vi "Calibartion-UI.vi"(8 "error in (no error)":errorcluster, 11 "Data (in)":T1={"Xml Path?"=path "", "Calib_List"=[], "Calibration Tbl Value"=-1, "Tbl_Size"=4294967295, "Parameter List"=[]}) -> (0 "error out":errorcluster, 3 "Data (out)":T1={"Xml Path?"=path "", "Calib_List"=[], "Calibration Tbl Value"=-1, "Tbl_Size"=4294967295, "Parameter List"=[]})   [LabVIEW 2010]
uses:
  Calibration_UI_Data.ctl
  Calibration dates.ctl
  <userlib>/_VIE Internal Reuse Library/_vie_lib_queued_message_handler.llb/VIE.Module.Queued Message Handler.enqueue.State.PolyChild.QueuedMessageHandler.vi
  <userlib>/_VIE Internal Reuse Library/_vie_lib_queued_message_handler.llb/VIE.Module.Queued Message Handler.[enqueue].State.PolyChild.QueuedMessageHandler.vi
  <vilib>/Utility/xml.llb/Write to XML File(string).vi
  <vilib>/Utility/xml.llb/Read From XML File(string).vi
  <userlib>/_VIE Internal Reuse Library/_vie_lib_queued_message_handler.llb/VIE.Module.Queued Message Handler.QueuedMessageHandler.dqGOOPClass.lvlib
panel:
  out "Cal Due Date":string="MM/DD/YY"
  in  "Calibration Details":i32(listbox)
  in  "Calibrate All":bool
  out "Name.Minor.Foreground":string="Automated Test Execution Software"
  out "Name.Major.Foreground":string="ATES"
  out "Name.Major.Background":string="ATES"
  out "Name.Minor.Background":string="Automated Test Execution Software"
  in  "Calibration Utility":bool
  out "IPG Calibration Status":bool
  # "(Double Click on the row to calibrate it)"
  # "Use the CVT as a data bus for data that is\nto be accesed outside of the VI.  It can be\nused for data passed around  inside the state\nmachine too, and all local data can be selectively\npurged from the CVT in the \"system.Exit\" state."
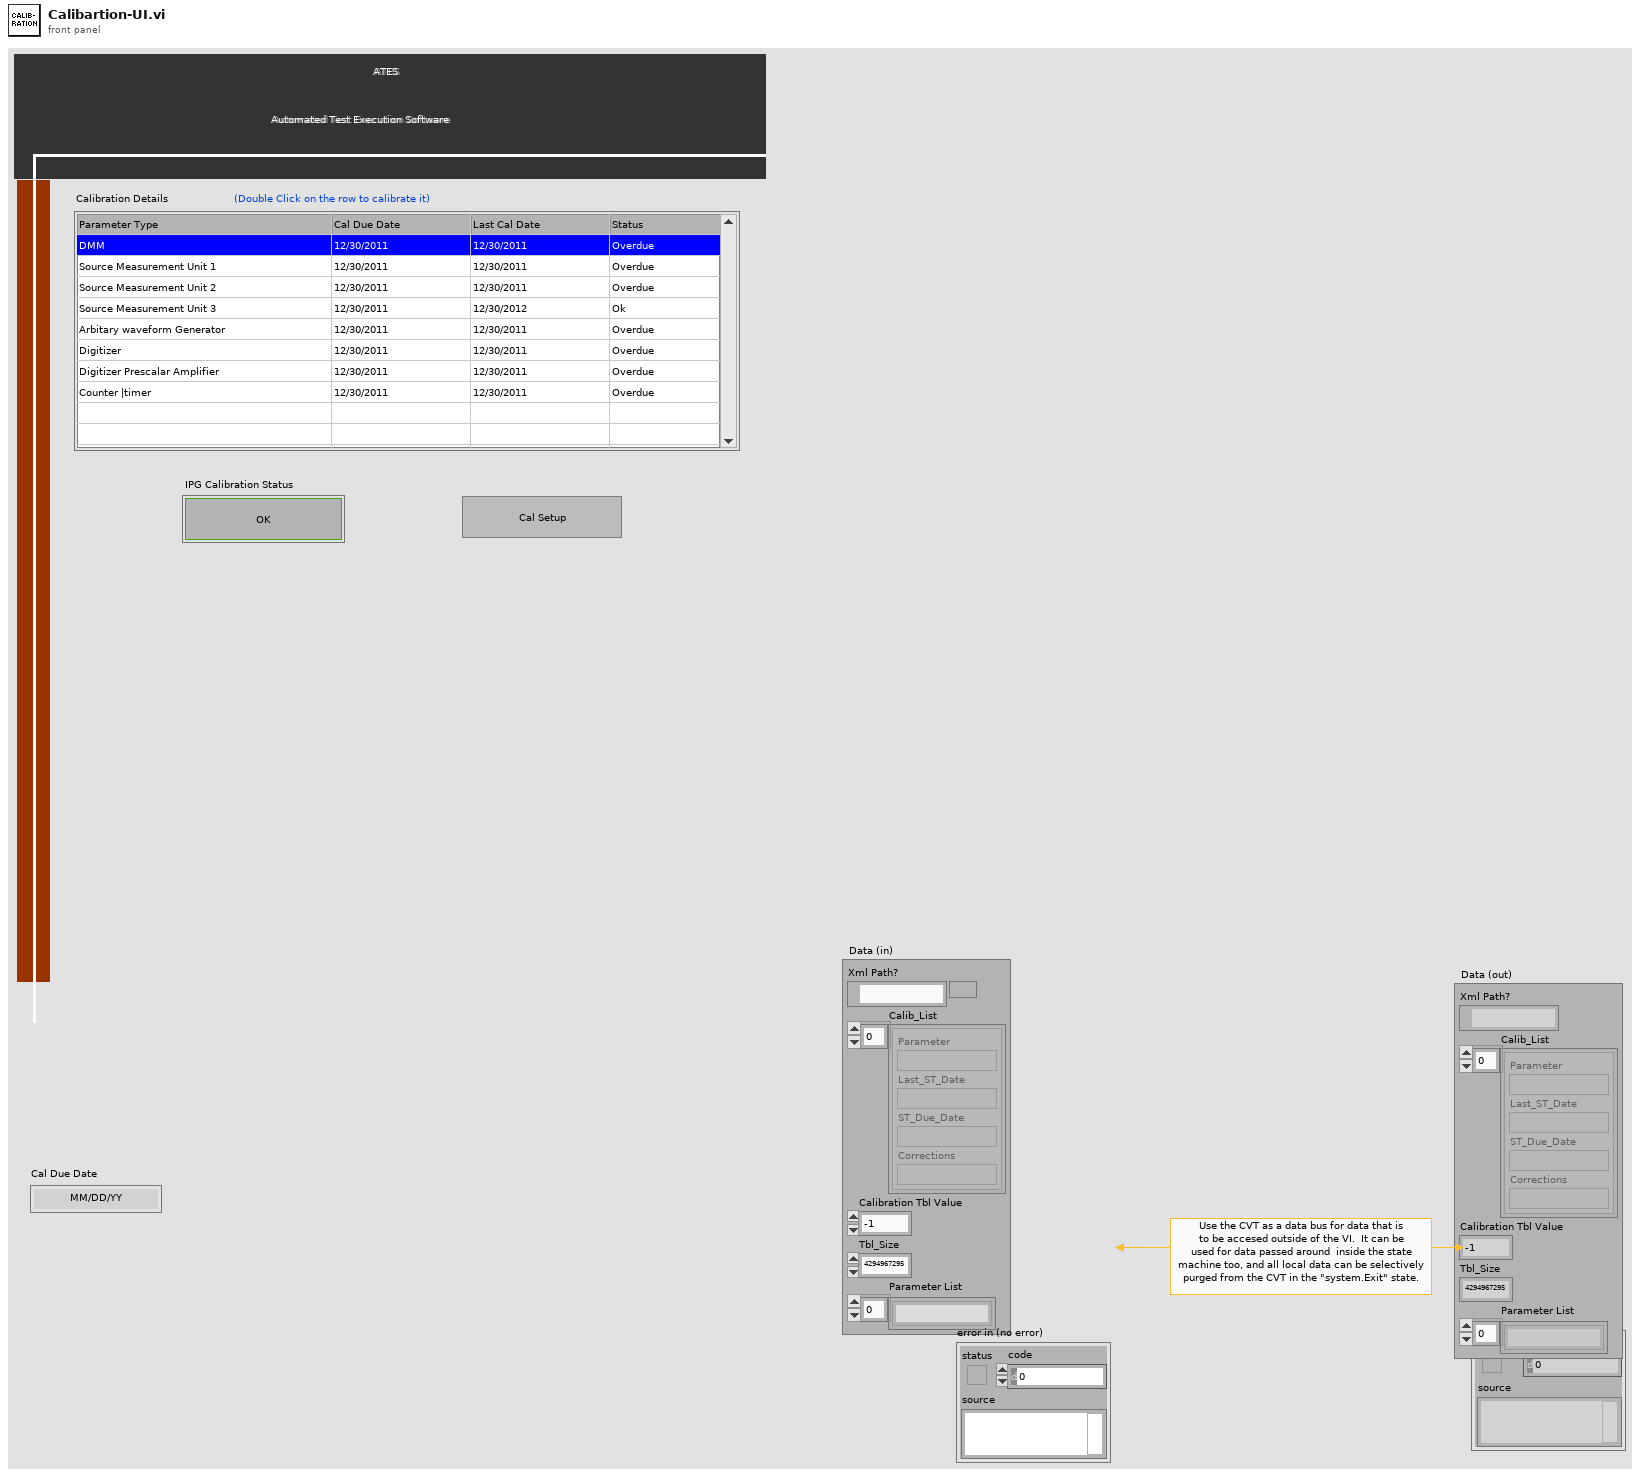
[diagram p1: front panel]
types:
  T1 = typedef "Calibration_UI_Data.ctl" = cluster{"Xml Path?":path, "Calib_List":T2[], "Calibration Tbl Value":i32, "Tbl_Size":u32, "Parameter List":string[]}
  T2 = typedef "Calibration dates.ctl" = cluster{"Parameter":string, "Last_ST_Date":string, "ST_Due_Date":string, "Corrections":string}
  T3 = enum16{"open", "replace", "create", "open or create", "replace or create", "replace or create with confirmation"}
  T4 = enum32{"invalid app kind", "Development System", "Run Time System", "Student Edition", "Embedded LabVIEW", "Evaluation", "Custom"}
  T5 = typedef "VIE.Module.Queued Message Handler.QueuedMessageHandler.dqGOOPClass.lvlib/VIE.Module.Queued Message Handler.dqClass_ObjectReference.ctl" = refnum<k1>
  T6 = typedef "LVPoint32TypeDef.ctl" = cluster{"Horizontal":i32, "Vertical":i32}
  T7 = typedef "LVRowAndColumnTypeDef.ctl" = cluster{"Row":i32, "Column":i32}
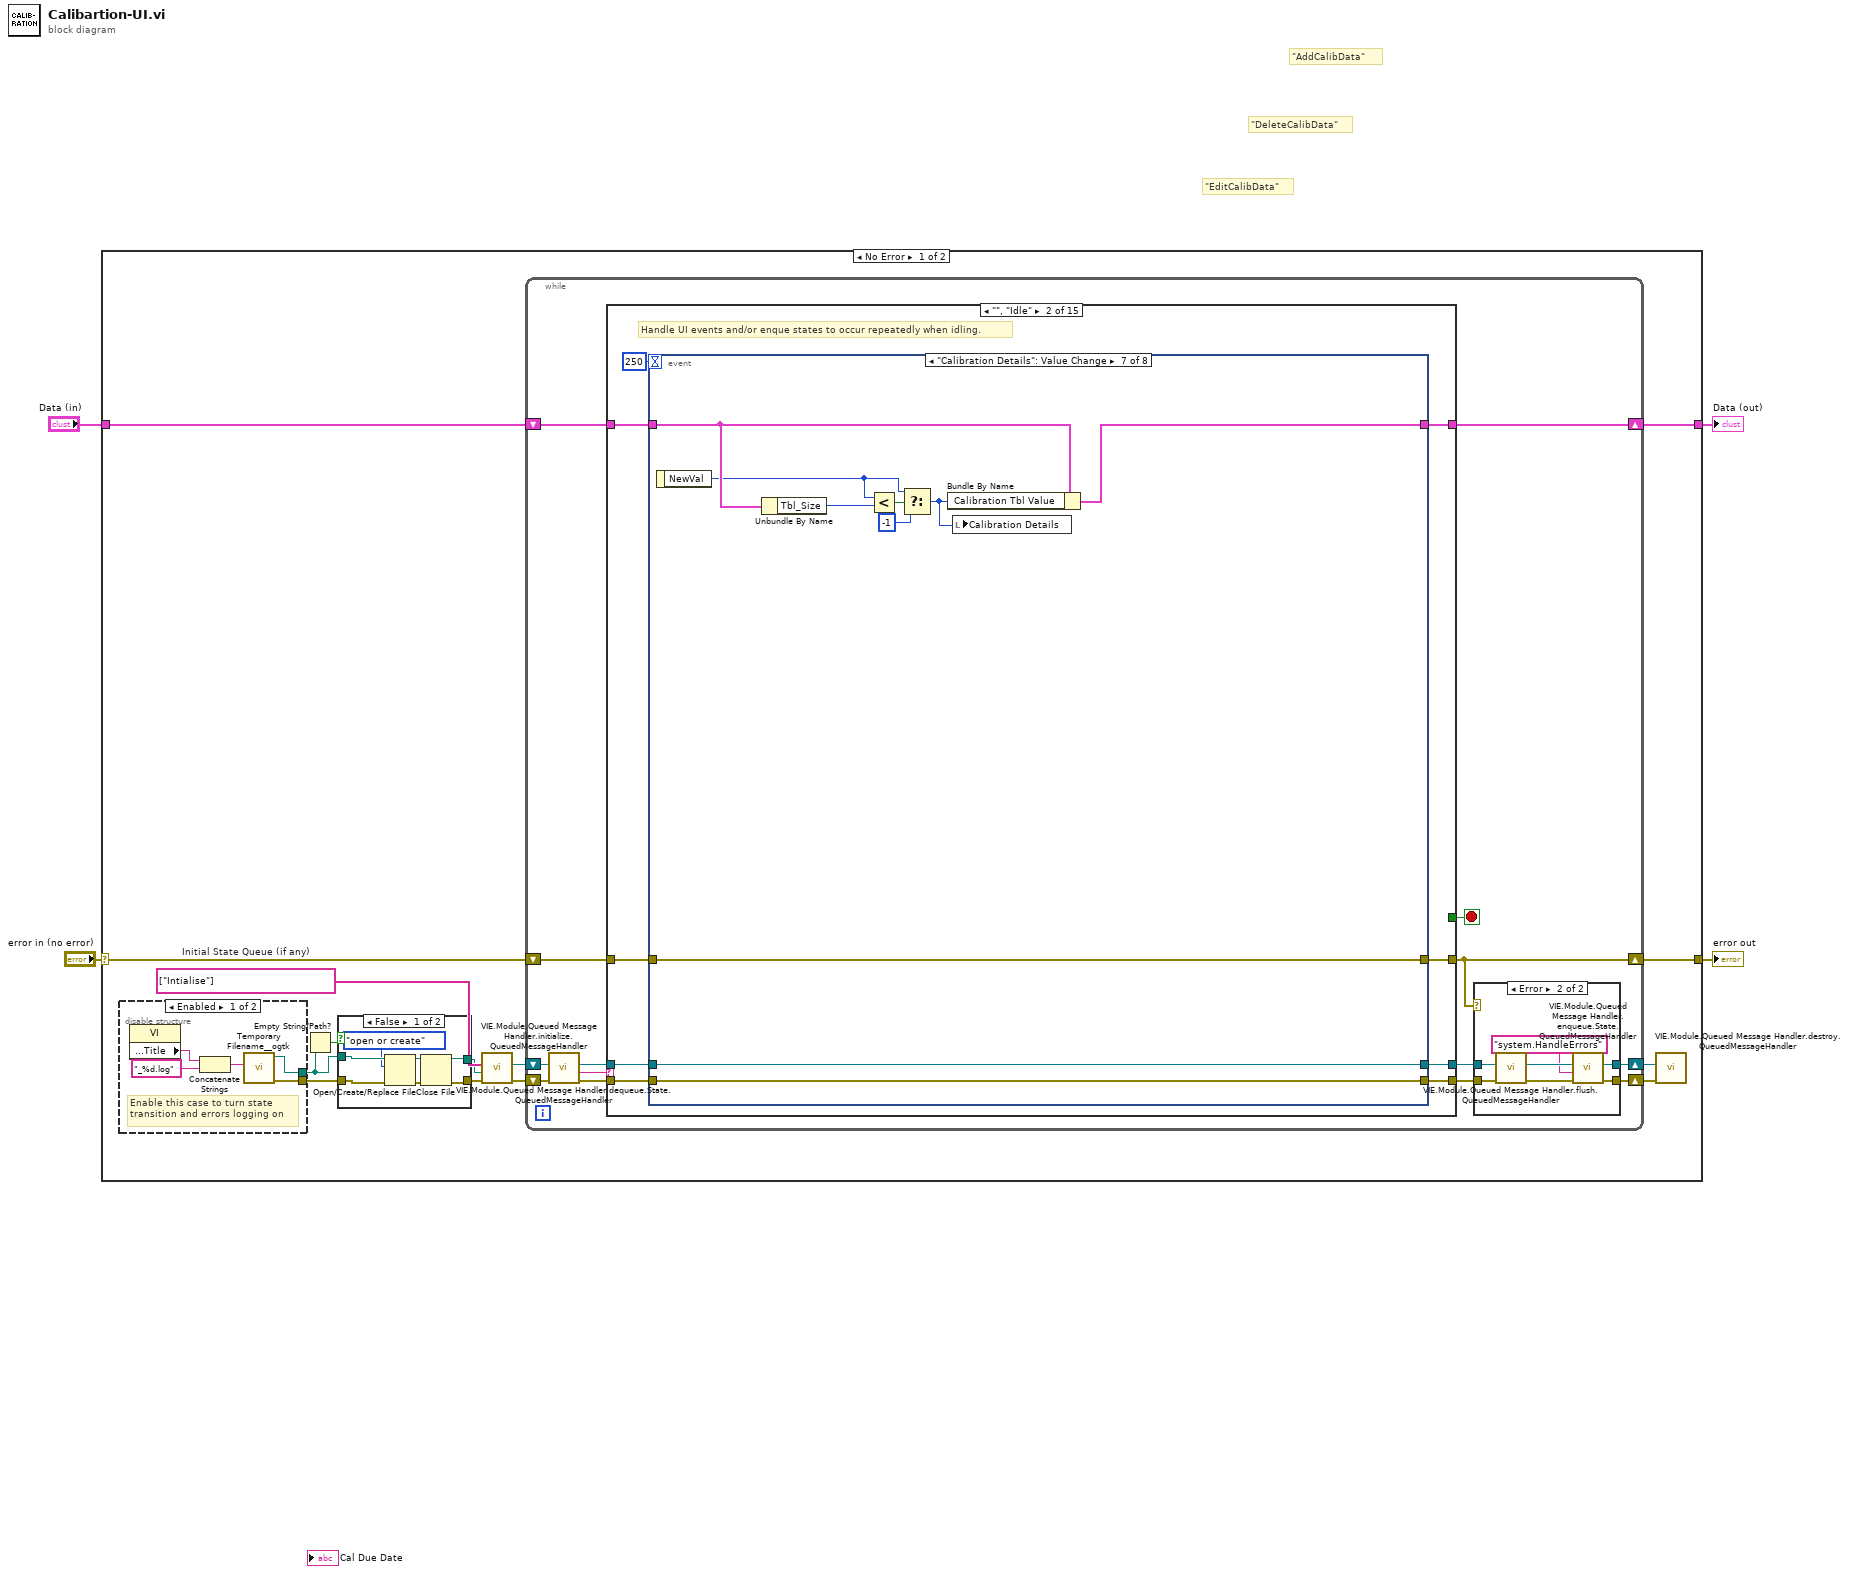
[diagram p0: block diagram]
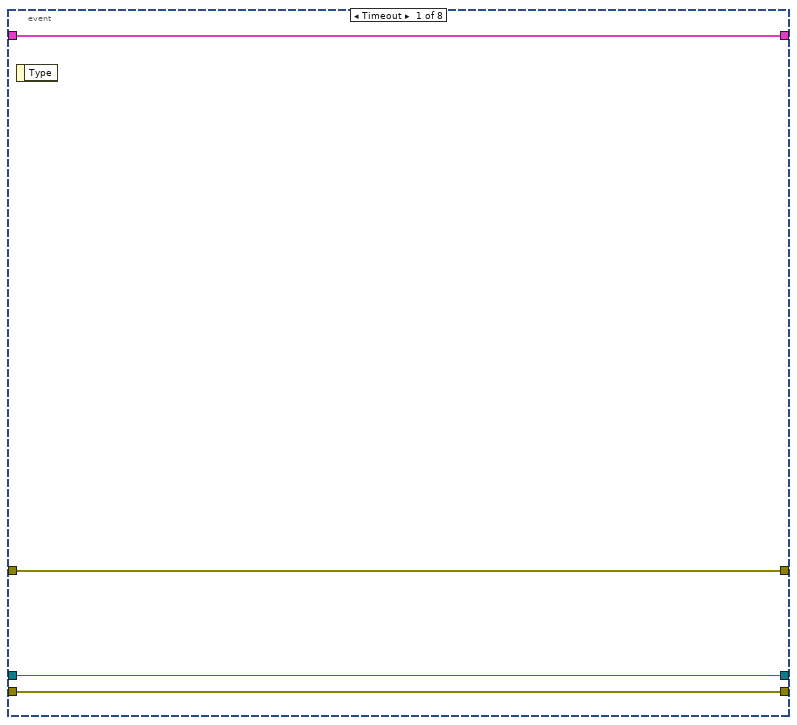
[diagram p6: hidden frame]
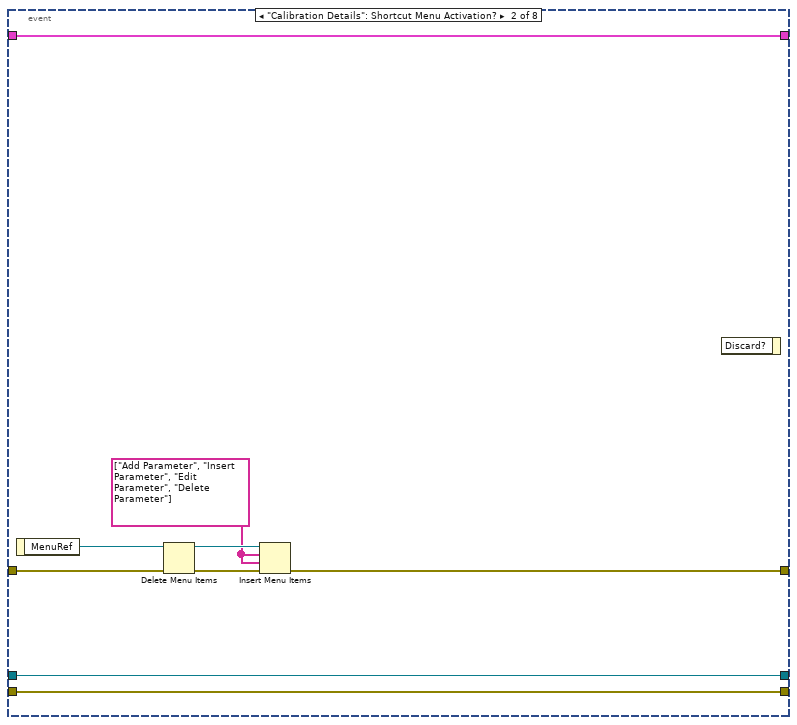
[diagram p7: hidden frame]
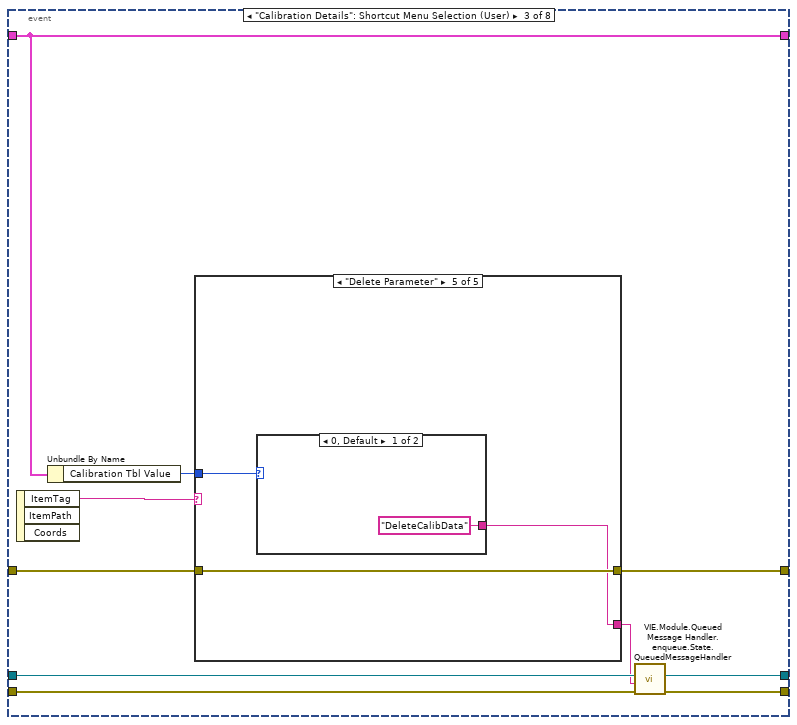
[diagram p8: hidden frame]
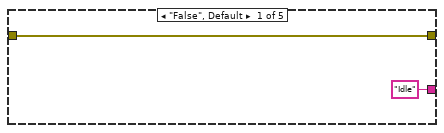
[diagram p9: hidden frame]
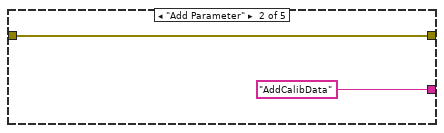
[diagram p10: hidden frame]
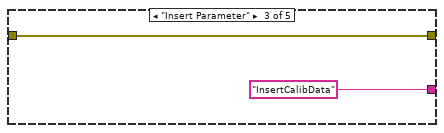
[diagram p11: hidden frame]
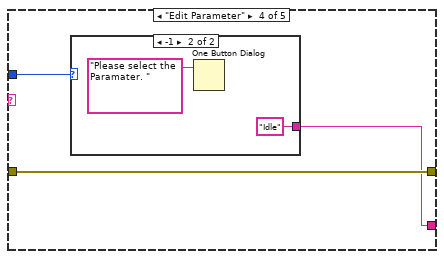
[diagram p12: hidden frame]
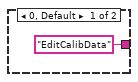
[diagram p13: hidden frame]
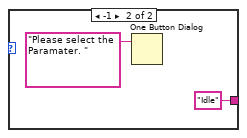
[diagram p14: hidden frame]
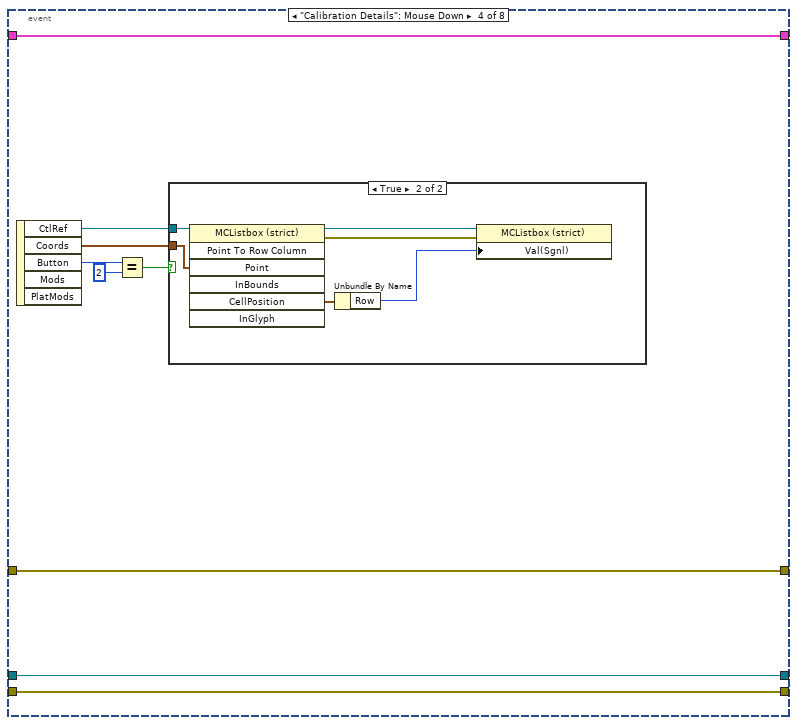
[diagram p15: hidden frame]
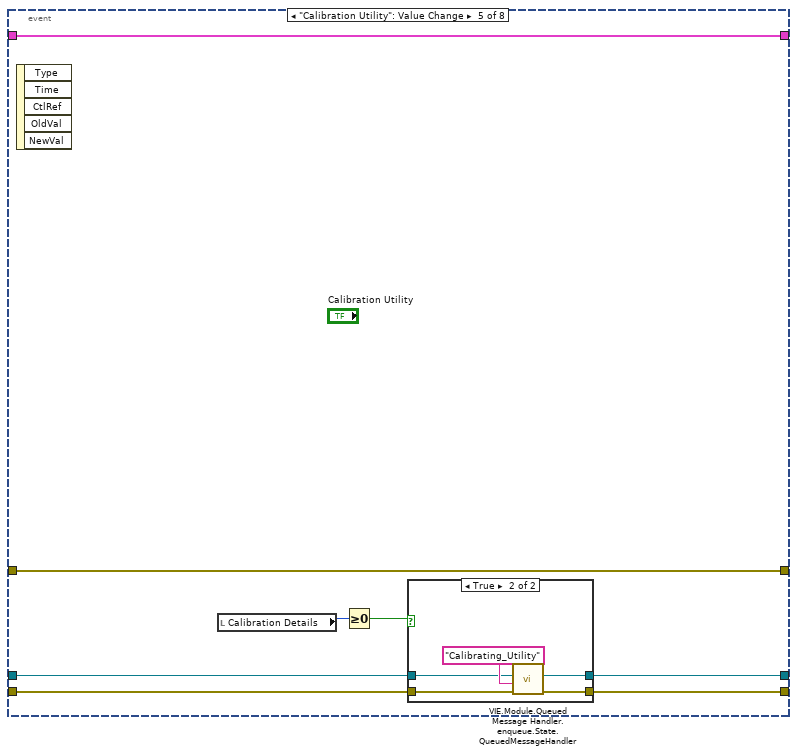
[diagram p17: hidden frame]
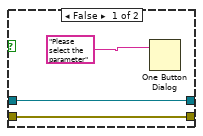
[diagram p18: hidden frame]
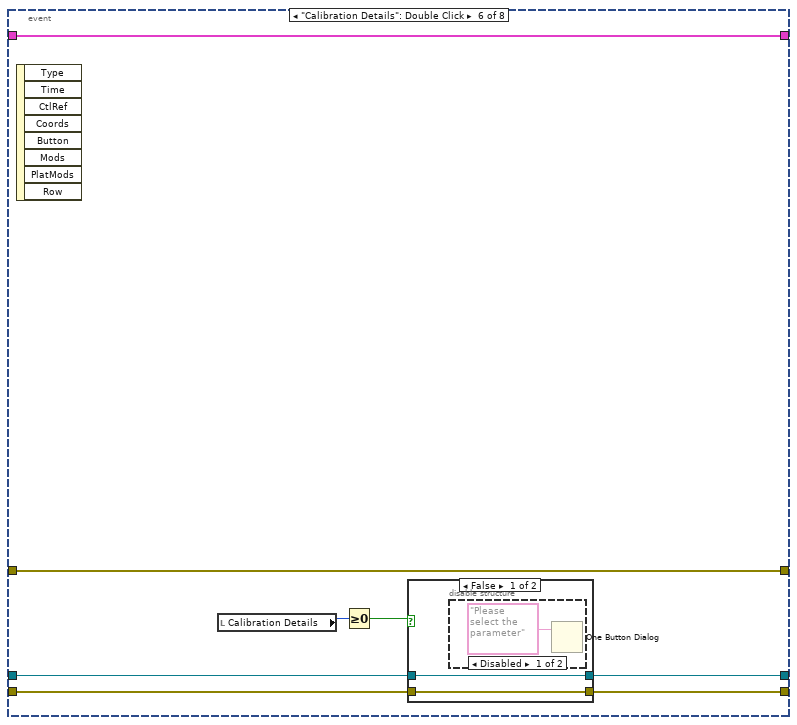
[diagram p19: hidden frame]
diagram:
  # "\"AddCalibData\""
  # "\"EditCalibData\""
  # "\"DeleteCalibData\""
  n1 = case shown="No Error" "error in (no error)" {
    selector: "error in (no error)" -> [w13 w462]
    tunnel: [w12 w462] -> w3
    tunnel: "Data (in)" -> [w10 w461]
    tunnel: [w14 w461] -> w1
    frame No Error {
      w11 = string[] ["Intialise"]  # Initial State Queue (if any)
      n2 = disable-structure shown="Enabled" {
        disable-tunnel: [w29 _] -> w8
        disable-tunnel: [w28 _] -> w9
        frame Enabled {
          # "Enable this case to turn state\ntransition and errors logging on"
          n3 = property class="VI"() -> ("Front Panel.Title"=w30:string)  [unwired: 2 in, 2 out]
          n4 = Concatenate Strings(w30, "_%d.log" ("string")) -> (w32:string)
          n5 = call <userlib>:"Temporary Filename__ogtk.vi"("pattern (lvtemp%d.tmp)"=w32) -> ("error out"=w29:errorcluster, "file in tmp dir"=w28:path)  [unwired: 5 in]
        }
        frame Disabled {
          # "Enable this case to turn state\ntransition and errors logging off"
        }
      }
      n6 = Empty String/Path?(string/path=w9) -> (empty?=w5:bool)
      n7 = case shown="False" w5 {
        tunnel: w8 -> [w25 w27]
        tunnel: [w20 w27] -> w7
        tunnel: w9 -> [w24 w26]
        tunnel: [w19 w26] -> w6
        frame False {
          n8 = Open/Create/Replace File(file path (use dialog)=w24, error in=w25, operation (0:open)=T3."open or create") -> (refnum out=w22:refnum<file>, error out=w21:errorcluster)  [unwired: 3 in, 1 out]
          n9 = Close File(refnum=w22, error in=w21) -> (path=w19:path, error out=w20:errorcluster)
        }
        frame True {
        }
      }
      n10 = call <userlib>:"VIE.Module.Queued Message Handler.initialize.QueuedMessageHandler.vi"("error in (no error)"=w7, "State Queue Log FilePath (\"\" = Do Not Log)"=w6, "Initial State Queue (empty)"=w11) -> ("error out"=w18:errorcluster, "QueuedMessageHandler.dqGOOPClass (out)"=w15:T5)  [unwired: 7 in]
      n11 = while {
        shift-right: [w35] -> w17
        shift-left: w18 -> [w43]
        shift-right: [w40] -> w14
        shift-left: w10 -> [w41]
        shift-right: [w38] -> w12
        shift-left: w13 -> [w39]
        shift-right: [w34] -> w16
        shift-left: w15 -> [w46]
        stop <- w33 stop-if-true
        n12 = call <userlib>:"VIE.Module.Queued Message Handler.dequeue.State.QueuedMessageHandler.vi"("error in (no error)"=w43, "QueuedMessageHandler.dqGOOPClass (in)"=w46) -> ("error out"=w44:errorcluster, "State Dequeued"=w42:string, "QueuedMessageHandler.dqGOOPClass (out)"=w45:T5)  [unwired: 7 in]
        n13 = case shown="\"\", \"Idle\"" w42 {
          selector: w42 -> [_ _ _ _ _ _ _ _ _ _ _ _ w413 _ _]
          tunnel: w44 -> [w56 w66 w179 w235 w267 w289 w314 w348 w371 w383 w400 w407 w412 w430 w454]
          tunnel: [w56 w61 w188 w247 w276 w300 w325 w356 w373 w381 w400 w407 w412 w421 w454] -> w37
          tunnel: w45 -> [w57 w65 w180 w236 w268 w290 w315 w350 w370 w384 w401 w408 w411 w431 w455]
          tunnel: [w57 w62 w187 w246 w275 w299 w324 w355 w372 w382 w401 w408 w411 w422 w455] -> w36
          tunnel: w41 -> [w59 w68 w183 w239 w271 w293 w318 w344 w368 w385 w392 w410 w420 w434 w453]
          tunnel: [w59 w64 w182 w238 w270 w292 w317 w344 w367 w385 w393 w410 w420 w434 w453] -> w40
          tunnel: w39 -> [w58 w67 w178 w245 w274 w298 w323 w354 w362 w379 w398 w409 w415 w432 w448]
          tunnel: [w58 w63 w186 w244 w273 w297 w322 w353 w357 w379 w397 w409 w414 w425 w447] -> w38
          tunnel: [_ _ _ _ _ _ _ _ _ _ _ _ _ _ TRUE] -> w33
          frame "---- Custom States --------------------------" {
            # "Do not put any code in here - this is a case divider, and is not a valid state, so any code here will not be executed."
          }
          frame "", "Idle" {
            # "Handle UI events and/or enque states to occur repeatedly when idling."
            n14 = event shown="[6] \"Calibration Details\": Value Change" {
              selector: _ -> [_ _ _ _ _ _ _ _]
              dyn-events: _ -> [_ _ _ _ _ _ _ _]
              timeout: 250 -> [_ _ _ _ _ _ _ _]
              tunnel: w68 -> [w72 w81 w83 w118 w132 w148 w162 w174]
              tunnel: w67 -> [w69 w74 w91 w115 w131 w147 w166 w173]
              tunnel: w66 -> [w70 w79 w88 w116 w130 w146 w165 w169]
              tunnel: w65 -> [w71 w80 w86 w117 w128 w144 w164 w171]
              tunnel: [w72 w81 w83 w118 w132 w148 w163 w174] -> w64
              tunnel: [w69 w73 w90 w115 w131 w147 w166 w173] -> w63
              tunnel: [w71 w80 w85 w117 w127 w143 w164 w170] -> w62
              tunnel: [w70 w79 w87 w116 w129 w145 w165 w168] -> w61
              event Timeout {
                n15 = event-data() -> ()  [unwired: 1 in, 1 out]
              }
              event "Calibration Details": Shortcut Menu Activation? {
                w75 = string[] ["Add Parameter", "Insert Parameter", "Edit Parameter", "Delete Parameter"]
                n16 = event-data() -> ("MenuRef"=w76:refnum<k9>)  [unwired: 1 in]
                n17 = Delete Menu Items(6:w74, 9:w76) -> (0:w77:errorcluster, 3:w78:refnum<k9>)  [unwired: 2 in]
                n18 = Insert Menu Items(6:w77, 7:w75, 8:w75, 9:w78) -> (0:w73:errorcluster)  [unwired: 2 in, 2 out]
                n19 = event-data() -> ()  [unwired: 2 in, 1 out]
              }
              event "Calibration Details": Shortcut Menu Selection (User) {
                n20 = event-data() -> ("ItemTag"=w89:string)  [unwired: 1 in, 2 out]
                n21 = Unbundle By Name(w83) -> ("Calibration Tbl Value"=w82:i32)
                n22 = case shown="\"Delete Parameter\"" w89 {
                  tunnel: w91 -> [w93 w95 w97 w100 w106]
                  tunnel: [w93 w95 w97 w100 w106] -> w90
                  tunnel: ["Idle" ("State to Enqueue") "AddCalibData" ("State to Enqueue") "InsertCalibData" ("State to Enqueue") w98 w104] -> w84
                  tunnel: w82 -> [_ _ _ w99 w105]
                  frame "False", Default {
                  }
                  frame "Add Parameter" {
                  }
                  frame "Insert Parameter" {
                  }
                  frame "Edit Parameter" {
                    n23 = case shown="-1" w99 {
                      tunnel: ["EditCalibData" ("State to Enqueue") "Idle" ("State to Enqueue")] -> w98
                      frame 0, Default {
                      }
                      frame -1 {
                        n24 = One Button Dialog(message="Please select the Paramater. ") -> ()  [unwired: 1 in, 1 out]
                      }
                    }
                  }
                  frame "Delete Parameter" {
                    n25 = case shown="0, Default" w105 {
                      tunnel: ["DeleteCalibData" ("State to Enqueue") "Idle" ("State to Enqueue")] -> w104
                      frame 0, Default {
                      }
                      frame -1 {
                        n26 = One Button Dialog(message="Please select the Paramater. ") -> ()  [unwired: 1 in, 1 out]
                      }
                    }
                  }
                }
                n27 = call-poly <userlib>:"VIE.Module.Queued Message Handler.enqueue.State.QueuedMessageHandler.vi"("error in (no error)"=w88, "State to Enqueue"=w84, "QueuedMessageHandler.dqGOOPClass (in)"=w86) -> ("error out"=w87:errorcluster, "QueuedMessageHandler.dqGOOPClass (out)"=w85:T5)  [unwired: 7 in]
              }
              event "Calibration Details": Mouse Down {
                n28 = event-data() -> ("CtlRef"=w112:refnum<vi>, "Coords"=w113:T6, "Button"=w111:u16)  [unwired: 1 in, 2 out]
                n29 = Equal?(x=w111, y=u16 2) -> (x = y?=w110:bool)
                n30 = case shown="True" w110 {
                  tunnel: w113 -> [_ w124]
                  tunnel: w112 -> [_ w123]
                  frame False {
                  }
                  frame True {
                    n31 = invoke class="MCListbox (strict)" method="Point To Row Column"(reference=w123, "Point"=w124) -> (reference out=w122:refnum<vi>, error out=w121:errorcluster, "CellPosition"=w120:T7)  [unwired: 5 in, 4 out]
                    n32 = Unbundle By Name(w120) -> ("Row"=w119:i32)
                    n33 = property class="MCListbox (strict)"(reference=w122, error in=w121, "Val(Sgnl)"=w119) -> ()  [unwired: 2 out]
                  }
                }
              }
              event "Calibration Utility": Value Change {
                n34 = event-data() -> ()  [unwired: 1 in, 5 out]
                n35 = local read "Calibration Details"() -> (w126:i32)
                n36 = Greater Or Equal To 0?(x=w126) -> (x >= 0?=w125:bool)
                n37 = case shown="True" w125 {
                  tunnel: w130 -> [w134 w139]
                  tunnel: [w134 w138] -> w129
                  tunnel: w128 -> [w135 w137]
                  tunnel: [w135 w136] -> w127
                  frame False {
                    n38 = One Button Dialog(message="Please select the parameter") -> ()  [unwired: 1 in, 1 out]
                  }
                  frame True {
                    n39 = call-poly <userlib>:"VIE.Module.Queued Message Handler.enqueue.State.QueuedMessageHandler.vi"("error in (no error)"=w139, "State to Enqueue"="Calibrating_Utility", "QueuedMessageHandler.dqGOOPClass (in)"=w137) -> ("error out"=w138:errorcluster, "QueuedMessageHandler.dqGOOPClass (out)"=w136:T5)  [unwired: 7 in]
                  }
                }
              }
              event "Calibration Details": Double Click {
                n40 = event-data() -> ()  [unwired: 1 in, 8 out]
                n41 = local read "Calibration Details"() -> (w142:i32)
                n42 = Greater Or Equal To 0?(x=w142) -> (x >= 0?=w141:bool)
                n43 = case shown="False" w141 {
                  tunnel: w146 -> [w149 w155]
                  tunnel: [w149 w154] -> w145
                  tunnel: w144 -> [w150 w153]
                  tunnel: [w150 w152] -> w143
                  frame False {
                    n44 = disable-structure shown="Disabled" {
                      frame Disabled {
                        n45 = One Button Dialog(message="Please select the parameter") -> ()  [unwired: 1 in, 1 out]
                      }
                      frame Enabled {
                      }
                    }
                  }
                  frame True {
                    n46 = call-poly <userlib>:"VIE.Module.Queued Message Handler.enqueue.State.QueuedMessageHandler.vi"("error in (no error)"=w155, "State to Enqueue"="Calibrating_Utility", "QueuedMessageHandler.dqGOOPClass (in)"=w153) -> ("error out"=w154:errorcluster, "QueuedMessageHandler.dqGOOPClass (out)"=w152:T5)  [unwired: 7 in]
                  }
                }
              }
              event "Calibration Details": Value Change {
                n47 = event-data() -> ("NewVal"=w158:i32)  [unwired: 1 in]
                n48 = Unbundle By Name(w162) -> ("Tbl_Size"=w161:u32)
                n49 = Less?(x=w158, y=w161) -> (x < y?=w160:bool)
                n50 = Select(t=w158, s=w160, f=-1) -> (s? t:f=w157:i32)
                n51 = Bundle By Name(cluster=w162, "Calibration Tbl Value"=w157) -> (w163:T1)
                n52 = local write "Calibration Details"(w157) -> ()
              }
              event Panel Close? {
                n53 = event-data() -> ()  [unwired: 1 in, 3 out]
                n54 = call-poly <userlib>:"VIE.Module.Queued Message Handler.enqueue.State.QueuedMessageHandler.vi"("error in (no error)"=w169, "State to Enqueue"="system.Exit", "QueuedMessageHandler.dqGOOPClass (in)"=w171) -> ("error out"=w168:errorcluster, "QueuedMessageHandler.dqGOOPClass (out)"=w170:T5)  [unwired: 7 in]
                n55 = event-data("Discard?"=TRUE) -> ()  [unwired: 1 in, 1 out]
              }
            }
          }
          frame "Calibrating_Utility" {
            n56 = Unbundle By Name(w183) -> ("Tbl_Size"=w177:u32, "Calib_List"=w184:T2[])
            n57 = Greater?(x=w177, y="Calibration Details") -> (0:w175:bool)
            n58 = case shown="False" w175 {
              tunnel: [w191 w203] -> w186
              tunnel: "Calibrate All" -> [_ w198]
              tunnel: w184 -> [_ w197]
              tunnel: w183 -> [w189 w196]
              tunnel: [w189 w195] -> w182
              tunnel: [string[] ["Idle"] w194] -> w181
              tunnel: w178 -> [w191 w193]
              tunnel: "Calibration Details" -> [_ w192]
              frame False {
              }
              frame True {
                n59 = Index Array(array=w197, index=w192) -> (element=w199:T2)
                n60 = call "Calibration Due date - UI.vi"("Calibration Info"=w199, "Calibrate All"=w198) -> ("Due Date"=w201:string, "Calibrated Date"=w200:string, "Modified"=w202:bool)  [unwired: 11 in]
                n61 = case shown="False" w202 {
                  tunnel: w193 -> [w205 w207]
                  tunnel: [w205 w207] -> w203
                  tunnel: w201 -> [_ w215]
                  tunnel: w200 -> [_ w214]
                  tunnel: w199 -> [_ w216]
                  tunnel: w198 -> [_ w217]
                  tunnel: w197 -> [_ w213]
                  tunnel: w192 -> [_ w212]
                  tunnel: w196 -> [w206 w211]
                  tunnel: [w206 w210] -> w195
                  tunnel: [string[] ["Idle"] string[] ["WriteCalData"]] -> w194
                  frame False {
                  }
                  frame True {
                    n62 = case shown="True" w217 {
                      tunnel: w216 -> [_ w232]
                      tunnel: w215 -> [w221 w231]
                      tunnel: w214 -> [w220 w230]
                      tunnel: w213 -> [w219 w229]
                      tunnel: w212 -> [_ w228]
                      tunnel: [w218 w226] -> w209
                      frame True {
                        n63 = for {
                          tunnel: w221 -> [w225]
                          tunnel: w220 -> [w224]
                          tunnel: w219 -> [w223] mode=indexing
                          tunnel: [w222] -> w218 mode=indexing
                          n64 = Bundle By Name(cluster=w223, "ST_Due_Date"=w225, "Last_ST_Date"=w224) -> (w222:T2)
                        }
                      }
                      frame False {
                        n65 = Bundle By Name(cluster=w232, "ST_Due_Date"=w231, "Last_ST_Date"=w230) -> (w227:T2)
                        n66 = Replace Array Subset(array=w229, new element=w227, index=w228) -> (w226:T2[])
                      }
                    }
                    n67 = Bundle By Name(cluster=w211, "Calib_List"=w209) -> (w210:T1)
                  }
                }
              }
            }
            n68 = call-poly <userlib>:"VIE.Module.Queued Message Handler.enqueue.State.QueuedMessageHandler.vi"("error in (no error)"=w179, "States to Enqueue"=w181, "QueuedMessageHandler.dqGOOPClass (in)"=w180) -> ("error out"=w188:errorcluster, "QueuedMessageHandler.dqGOOPClass (out)"=w187:T5)  [unwired: 7 in]
          }
          frame "EditCalibData" {
            n69 = Unbundle By Name(w239) -> ("Calib_List"=w240:T2[], "Calibration Tbl Value"=w234:i32)  [unwired: 1 out]
            n70 = Index Array(array=w240, index=w234) -> (element=w241:T2)
            n71 = call "Calibration Parameter Add_Modify - UI.vi"("Add??"=FALSE, "Parameter Details In"=w241) -> ("Processed"=w243:bool, "Parameter Details Out"=w242:T2)  [unwired: 7 in, 1 out]
            n72 = case shown="True" w243 {
              tunnel: w245 -> [w249 w252]
              tunnel: [w249 w252] -> w244
              tunnel: w242 -> [_ w251]
              tunnel: w240 -> [_ w258]
              tunnel: w234 -> [_ w257]
              tunnel: w239 -> [w250 w256]
              tunnel: [w250 w255] -> w238
              tunnel: [string[] ["Idle"] string[] ["WriteCalData"]] -> w237
              frame False {
              }
              frame True {
                n73 = Replace Array Subset(array=w258, new element=w251, index=w257) -> (w254:T2[])
                n74 = Bundle By Name(cluster=w256, "Calib_List"=w254) -> (w255:T1)
              }
            }
            n75 = call-poly <userlib>:"VIE.Module.Queued Message Handler.enqueue.State.QueuedMessageHandler.vi"("error in (no error)"=w235, "States to Enqueue"=w237, "QueuedMessageHandler.dqGOOPClass (in)"=w236) -> ("error out"=w247:errorcluster, "QueuedMessageHandler.dqGOOPClass (out)"=w246:T5)  [unwired: 7 in]
          }
          frame "DeleteCalibData" {
            n76 = Unbundle By Name(w271) -> ("Calib_List"=w272:T2[], "Calibration Tbl Value"=w266:i32)
            n77 = Index Array(array=w272, index=w266) -> (element=w265:T2)
            n78 = Unbundle By Name(w265) -> ("Parameter"=w264:string)
            n79 = Concatenate Strings("Do you want to delete " ("string"), w264, " ?" ("string")) -> (w261:string)
            n80 = Two Button Dialog(message=w261, 2:"Delete" ("T button name (\"OK\")")) -> (T button?=w259:bool)  [unwired: 1 in]
            n81 = case shown="True" w259 {
              tunnel: w274 -> [w278 w281]
              tunnel: [w278 w281] -> w273
              tunnel: w272 -> [_ w286]
              tunnel: w271 -> [w279 w285]
              tunnel: [w279 w284] -> w270
              tunnel: [string[] ["Idle"] string[] ["WriteCalData"]] -> w269
              tunnel: w266 -> [_ w280]
              frame False {
              }
              frame True {
                n82 = Delete From Array(array=w286, index=w280) -> (array with subset deleted=w283:T2[])  [unwired: 1 in, 1 out]
                n83 = Bundle By Name(cluster=w285, "Calib_List"=w283) -> (w284:T1)
              }
            }
            n84 = call-poly <userlib>:"VIE.Module.Queued Message Handler.enqueue.State.QueuedMessageHandler.vi"("error in (no error)"=w267, "States to Enqueue"=w269, "QueuedMessageHandler.dqGOOPClass (in)"=w268) -> ("error out"=w276:errorcluster, "QueuedMessageHandler.dqGOOPClass (out)"=w275:T5)  [unwired: 7 in]
          }
          frame "AddCalibData" {
            n85 = Unbundle By Name(w293) -> ("Calib_List"=w294:T2[], "Parameter List"=w288:string[])
            n86 = call "Calibration Parameter Add_Modify - UI.vi"("Parameter List"=w288, "Add??"=TRUE) -> ("Processed"=w296:bool, "Parameter Details Out"=w295:T2)  [unwired: 7 in, 1 out]
            n87 = case shown="True" w296 {
              tunnel: w298 -> [w302 w305]
              tunnel: [w302 w305] -> w297
              tunnel: w295 -> [_ w304]
              tunnel: w294 -> [_ w310]
              tunnel: w293 -> [w303 w309]
              tunnel: [w303 w308] -> w292
              tunnel: [string[] ["Idle"] string[] ["WriteCalData"]] -> w291
              frame False {
              }
              frame True {
                n88 = Build Array (concatenate)(w310, w304) -> (w307:T2[])
                n89 = Bundle By Name(cluster=w309, "Calib_List"=w307) -> (w308:T1)
              }
            }
            n90 = call-poly <userlib>:"VIE.Module.Queued Message Handler.enqueue.State.QueuedMessageHandler.vi"("error in (no error)"=w289, "States to Enqueue"=w291, "QueuedMessageHandler.dqGOOPClass (in)"=w290) -> ("error out"=w300:errorcluster, "QueuedMessageHandler.dqGOOPClass (out)"=w299:T5)  [unwired: 7 in]
          }
          frame "InsertCalibData" {
            n91 = Unbundle By Name(w318) -> ("Calibration Tbl Value"=w313:i32, "Calib_List"=w319:T2[], "Parameter List"=w312:string[])
            n92 = call "Calibration Parameter Add_Modify - UI.vi"("Parameter List"=w312, "Add??"=TRUE) -> ("Processed"=w321:bool, "Parameter Details Out"=w320:T2)  [unwired: 7 in, 1 out]
            n93 = case shown="True" w321 {
              tunnel: w323 -> [w327 w331]
              tunnel: [w327 w331] -> w322
              tunnel: w320 -> [_ w330]
              tunnel: w319 -> [_ w336]
              tunnel: w318 -> [w328 w335]
              tunnel: [w328 w334] -> w317
              tunnel: [string[] ["Idle"] string[] ["WriteCalData"]] -> w316
              tunnel: w313 -> [_ w329]
              frame False {
              }
              frame True {
                n94 = case shown="0, Default" w329 {
                  selector: w329 -> [w338 _]
                  tunnel: w336 -> [w340 w343]
                  tunnel: [w337 w342] -> w333
                  tunnel: w330 -> [w339 w341]
                  frame 0, Default {
                    n95 = Insert Into Array(array=w340, index=w338, new element=w339) -> (w337:T2[])
                  }
                  frame -1 {
                    n96 = Build Array (concatenate)(w343, w341) -> (w342:T2[])
                  }
                }
                n97 = Bundle By Name(cluster=w335, "Calib_List"=w333) -> (w334:T1)
              }
            }
            n98 = call-poly <userlib>:"VIE.Module.Queued Message Handler.enqueue.State.QueuedMessageHandler.vi"("error in (no error)"=w314, "States to Enqueue"=w316, "QueuedMessageHandler.dqGOOPClass (in)"=w315) -> ("error out"=w325:errorcluster, "QueuedMessageHandler.dqGOOPClass (out)"=w324:T5)  [unwired: 7 in]
          }
          frame "WriteCalData" {
            n99 = Unbundle By Name(w344) -> ("Xml Path?"=w352:path, "Calib_List"=w345:T2[])
            n100 = Flatten To XML(anything=w345) -> (xml string=w346:string)
            n101 = call-poly <vilib>:"Write to XML File.vi"("error in (no error)"=w354, "XML Input"=w346, "XML File Path"=w352) -> ("error out"=w353:errorcluster)  [unwired: 6 in, 2 out]
            n102 = call <userlib>:"VIE.Module.Queued Message Handler.flush.QueuedMessageHandler.vi"("error in (no error)"=w348, "QueuedMessageHandler.dqGOOPClass (in)"=w350) -> ("error out"=w347:errorcluster, "QueuedMessageHandler.dqGOOPClass (out)"=w349:T5)  [unwired: 7 in, 1 out]
            n103 = call-poly <userlib>:"VIE.Module.Queued Message Handler.enqueue.State.QueuedMessageHandler.vi"("error in (no error)"=w347, "States to Enqueue"=string[] ["ReadCalData"], "QueuedMessageHandler.dqGOOPClass (in)"=w349) -> ("error out"=w356:errorcluster, "QueuedMessageHandler.dqGOOPClass (out)"=w355:T5)  [unwired: 7 in]
          }
          frame "Intialise" {
            (unwired) string[] ["DMM", "Source Measurement Unit 1", "Source Measurement Unit 2", "Source Measurement Unit 3", "Arbitary waveform Generator", "Digitizer", "Digitizer Prescalar Amplifier", "Counter |timer"] ("Parameter_List")
            w364 = "Calibration" ("Name.Minor.Background")
            w365 = "QIG-IPG Tester" ("Name.Major.Background")
            # "c:\\IPG test builds\\data\\station calibration file.xml"
            # "Intialises the data"
            n104 = call <userlib>:"Fit VI window to Largest Dec__ogtk.vi"("error in (no error)"=w362) -> ("error out"=w358:errorcluster)  [unwired: 5 in, 1 out]
            n105 = disable-structure shown="Enabled" {
              disable-tunnel: [w374 path "c:/IPG test builds/data/station calibration file.xml" ("appended path")] -> w366
              frame Disabled {
                n106 = Current VI's Path() -> (path=w377:path)
                n107 = Strip Path(path=w377) -> (stripped path=w376:path)  [unwired: 1 out]
                n108 = Build Path(base path=w376, name or relative path="station calibration file.xml") -> (appended path=w374:path)
              }
              frame Enabled {
              }
            }
            n109 = local write "Calibrate All"(FALSE ("Calibrate All")) -> ()
            n110 = call "Check and Create XML.vi"("Path In"=w366) -> ("Path Out"=w360:path)  [unwired: 9 in, 1 out]
            n111 = property on="Calibration Details" class="MCListbox (strict)"(error in=w358, "ColHdrString"=string[] ["Parameter Type", "Cal Due Date", "Last Cal Date", "Status"], "ItemNames"=string[][] [] ("Item Names")) -> (error out=w357:errorcluster)  [unwired: 1 in, 1 out]
            n112 = Bundle By Name(cluster=w368, "Xml Path?"=w360) -> (w367:T1)
            n113 = call-poly <userlib>:"VIE.Module.Queued Message Handler.enqueue.State.QueuedMessageHandler.vi"("error in (no error)"=w371, "States to Enqueue"=string[] ["ReadCalData", "Idle"], "QueuedMessageHandler.dqGOOPClass (in)"=w370) -> ("error out"=w373:errorcluster, "QueuedMessageHandler.dqGOOPClass (out)"=w372:T5)  [unwired: 7 in]
            "Name.Minor.Background" <- w364
            "Name.Major.Background" <- w365
            "Name.Major.Foreground" <- w365
            "Name.Minor.Foreground" <- w364
          }
          frame "custom.CleanUp" {
            # "Put code in this state that sets/resets system to a safe state, if required."
            n114 = call-poly <userlib>:"VIE.Module.Queued Message Handler.enqueue.State.QueuedMessageHandler.vi"("error in (no error)"=w383, "State to Enqueue"="system.Exit", "QueuedMessageHandler.dqGOOPClass (in)"=w384) -> ("error out"=w381:errorcluster, "QueuedMessageHandler.dqGOOPClass (out)"=w382:T5)  [unwired: 7 in]
          }
          frame "ReadCalData" {
            # "Put code in this state that sets/resets system to a safe state, if required."
            n115 = Unbundle By Name(w392) -> ("Xml Path?"=w391:path)
            n116 = call-poly <vilib>:"Read From XML File.vi"("error in (no error)"=w398, "XML File Path"=w391) -> ("error out"=w397:errorcluster, "XML Elements"=w399:string)  [unwired: 7 in, 1 out]
            n117 = Unflatten From XML(xml string=w399, type=T2[] []) -> (value=w390:T2[])  [unwired: 1 in, 1 out]
            n118 = call "Check Cal Dates.vi"("Calibration List"=w390) -> ("Status"=w394:string[], "Calibration Status"=→"IPG Calibration Status":bool)  [unwired: 9 in]
            n119 = for {
              tunnel: w390 -> [w406] mode=indexing
              tunnel: [w404] -> w388 mode=indexing
              tunnel: w394 -> [w405] mode=indexing
              n120 = Cluster To Array(cluster=w406) -> (array=w403:string[])
              n121 = Delete From Array(array=w403) -> (array with subset deleted=w402:string[])  [unwired: 2 in, 1 out]
              n122 = Build Array (concatenate)(w402, w405) -> (w404:string[])
            }
            n123 = Array Size(array=w390) -> (size(s)=w389:i32)
            n124 = Index Array(array=w388, index (col)=0 ("disabled index (col)")) -> (element=w386:string[])  [unwired: 1 in]
            n125 = property on="Calibration Details" class="MCListbox (strict)"("ItemNames"=w388) -> ()  [unwired: 2 in, 2 out]
            n126 = Bundle By Name(cluster=w392, "Calib_List"=w390, "Tbl_Size"=w389, "Parameter List"=w386) -> (w393:T1)
          }
          frame "---- System States --------------------------" {
            # "Do not put any code in here - this is a case divider, and is not a valid state, so any code here will not be executed."
          }
          frame "system.StateNameSyntaxError", Default {
            # "Do not alter the code in here - this is a system state that is required by the state machine architecture."
            n127 = property class="VI"() -> ("Name"=w416:string)  [unwired: 2 in, 2 out]
            n128 = Format Into String(format string="Syntax Error - Requested State not found in State Machine Architecture.\n\nArchitecture: %s\nState Requested: %s", w416, w413) -> (resulting string=w417:string)  [unwired: 2 in, 1 out]
            n129 = call <vilib>:"Error Cluster From Error Code.vi"("error in (no error)"=w415, "error message (\"\")"=w417, "error code (0)"=46) -> ("error out"=w414:errorcluster)  [unwired: 6 in]
          }
          frame "system.HandleErrors" {
            # "Do not alter the code in here - this is a system state that is required by the state machine architecture."
            # "Handle errors by presenting a dialog box to the\nuser and logging the error to file (if enabled)"
            n130 = call <vilib>:"Simple Error Handler.vi"("error in (no error)"=w432) -> ("code out"=w428:i32, "source out"=w427:string, "error out"=w429:errorcluster)  [unwired: 4 in, 2 out]
            n131 = Format Into String(format string="ERROR: Code=%d, Source=\"%s\"", w428, w427) -> (resulting string=w426:string)  [unwired: 2 in, 1 out]
            n132 = call <vilib>:"Clear Errors.vi"("error in (no error)"=w429) -> ("error out"=w425:errorcluster)  [unwired: 6 in]
            n133 = call <userlib>:"VIE.Module.Queued Message Handler.logEvent.QueuedMessageHandler.vi"("error in (no error)"=w430, "Event to Log"=w426, "QueuedMessageHandler.dqGOOPClass (in)"=w431) -> ("error out"=w423:errorcluster, "QueuedMessageHandler.dqGOOPClass (out)"=w424:T5)  [unwired: 7 in]
            n134 = disable-structure shown="Enabled" {
              disable-tunnel: w424 -> [w439 w444 w445]
              disable-tunnel: w423 -> [w438 w443 w446]
              disable-tunnel: [w437 w442 w445] -> w422
              disable-tunnel: [w436 w441 w446] -> w421
              frame Disabled {
                # "Enable this case to force software\nto exit on error."
                n135 = call-poly <userlib>:"VIE.Module.Queued Message Handler.enqueue.State.QueuedMessageHandler.vi"("error in (no error)"=w438, "State to Enqueue"="system.Exit", "QueuedMessageHandler.dqGOOPClass (in)"=w439) -> ("error out"=w436:errorcluster, "QueuedMessageHandler.dqGOOPClass (out)"=w437:T5)  [unwired: 7 in]
              }
              frame Enabled {
                # "Enable this case to force software\nto cleanup then exit on error."
                n136 = call-poly <userlib>:"VIE.Module.Queued Message Handler.enqueue.State.QueuedMessageHandler.vi"("error in (no error)"=w443, "States to Enqueue"=string[] ["custom.CleanUp", "system.Exit"], "QueuedMessageHandler.dqGOOPClass (in)"=w444) -> ("error out"=w441:errorcluster, "QueuedMessageHandler.dqGOOPClass (out)"=w442:T5)  [unwired: 7 in]
              }
              frame Disabled {
                # "Enable this case to force software\nto continue on error."
              }
            }
          }
          frame "system.Exit" {
            # "Do not alter the code in here - this is a system state that is required by the state machine architecture."
            n137 = property class="App"(error in=w448) -> (error out=w449:errorcluster, "App.Kind"=w452:T4)  [unwired: 1 in, 1 out]
            n138 = Equal?(x=w452, y=T4."Development System") -> (x = y?=w450:bool)
            n139 = case shown="False" w450 {
              tunnel: w449 -> [w459 w460]
              tunnel: [w458 w460] -> w447
              frame False {
                n140 = control-ref of="This VI"() -> (w457:refnum<vi>)
                n141 = invoke class="VI" method="FP.Close"(reference=w457, error in=w459) -> (error out=w458:errorcluster)  [unwired: 1 in, 2 out]
              }
              frame True {
              }
            }
          }
        }
        n142 = case shown="Error" w38 {
          tunnel: w37 -> [w47 w53]
          tunnel: w36 -> [w48 w52]
          tunnel: [w47 w51] -> w35
          tunnel: [w48 w50] -> w34
          frame No Error {
          }
          frame Error {
            n143 = call <userlib>:"VIE.Module.Queued Message Handler.flush.QueuedMessageHandler.vi"("error in (no error)"=w53, "QueuedMessageHandler.dqGOOPClass (in)"=w52) -> ("error out"=w55:errorcluster, "QueuedMessageHandler.dqGOOPClass (out)"=w54:T5)  [unwired: 7 in, 1 out]
            n144 = call-poly <userlib>:"VIE.Module.Queued Message Handler.enqueue.State.QueuedMessageHandler.vi"("error in (no error)"=w55, "State to Enqueue"="system.HandleErrors", "QueuedMessageHandler.dqGOOPClass (in)"=w54) -> ("error out"=w51:errorcluster, "QueuedMessageHandler.dqGOOPClass (out)"=w50:T5)  [unwired: 7 in]
          }
        }
      }
      n145 = call <userlib>:"VIE.Module.Queued Message Handler.destroy.QueuedMessageHandler.vi"("error in (no error)"=w17, "QueuedMessageHandler.dqGOOPClass (in)"=w16) -> ()  [unwired: 9 in, 1 out]
    }
    frame Error {
      # "An error was passed into the VI, so do not execute and pass the error and input CVT out."
    }
  }
  "error out" <- w3
  "Data (out)" <- w1
